vi "Teleop.vi"(10 "Match Info":T1={"Autonomous Elapsed Seconds"=0.0, "TeleOp Elapsed Seconds"=0.0, "Disabled Elapsed Seconds"=0.0, "Visited Autonomous"=FALSE, "Visited TeleOp"=FALSE, "Visited Disabled"=FALSE, "Autonomous Settings"={"Autonomous Style"=enum."Independent", "VI Refnum"=refnum}}, 11 "Call Context":T2) -> ()   [LabVIEW 2013]
doc: "This VI is called for each TeleOp packet received from the DS where the robot is not disabled. It is often used to read from the joysticks and update I/O or to update setpoints for timed control loops. It should complete and return within 20 milliseconds or it may miss DS packets."
uses:
  <vilib>/Rock Robotics/WPI/DriverStation/WPI_DriverStationDerivedRobotMode.ctl
  <vilib>/Rock Robotics/WPI/DriverStation/WPI_DriverStationMatch Info.ctl
  Robot Global Data.vi
  <vilib>/Rock Robotics/WPI/Solenoid/Deprecated/WPI_SolenoidSetBool.vi
  <vilib>/Rock Robotics/WPI/Joystick/WPI_JoystickGetSetRefNum.vi
  <vilib>/Rock Robotics/WPI/Solenoid/Deprecated/WPI_SolenoidGetBool.vi
  <vilib>/Rock Robotics/WPI/RobotDrive/WPI_RobotDriveGetSetRefNum.vi
panel:
  in  "Shoulder Limit":dbl=5.0
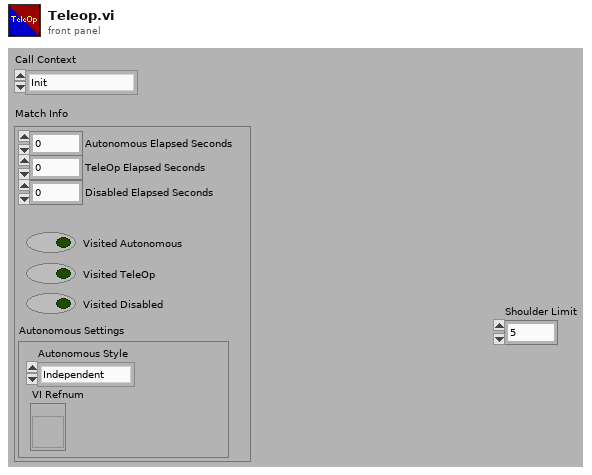
[diagram p1: front panel]
types:
  T1 = typedef "WPI_DriverStationMatch Info.ctl" = cluster{"Autonomous Elapsed Seconds":dbl, "TeleOp Elapsed Seconds":dbl, "Disabled Elapsed Seconds":dbl, "Visited Autonomous":bool, "Visited TeleOp":bool, "Visited Disabled":bool, "Autonomous Settings":cluster{"Autonomous Style":enum16{"Iterative", "Independent"}, "VI Refnum":refnum<vi>}}
  T2 = typedef "WPI_DriverStationDerivedRobotMode.ctl" = enum16{"Init", "Execute", "Stop"}
  T3 = typedef "WPI_JoystickDevRef.ctl" = cluster{"Device":T4}
  T4 = typedef "WPI_JoystickDeviceEnum.ctl" = enum16{"USB 1", "USB 2", "USB 3", "USB 4", "Kinect 1", "Kinect 2"}
  T5 = typedef "WPI_RobotDriveDevRef.ctl" = cluster{"DevStatus":errorcluster, "Motors[]":T6[], "Square Inputs":bool, "Max Output":dbl, "Isochronous":bool}
  T6 = typedef "WPI_MotorControlDeviceRef.ctl" = cluster{"DeviceStatus":errorcluster, "Type":enum16{"PWM", "CAN"}, "PWM":cluster{"Digital Module":T7, "PWM Channel":T8, "DeadBand":T9}, "CAN":cluster{"Device Number":u8, "Control Mode":T10, "Semaphore":T11, "Max Vout":dbl}, "Invert":bool, "TransformRef":T12, "InvTransformRef":T12}
  T7 = typedef "FPGA_TypedefDigitalModule.ctl" = enum16{"Digital Module 1", "Digital Module 2"}
  T8 = typedef "FPGA_DIOPWMChannel.ctl" = enum8{"PWM 1", "PWM 2", "PWM 3", "PWM 4", "PWM 5", "PWM 6", "PWM 7", "PWM 8", "PWM 9", "PWM 10", "Invalid"}
  T9 = typedef "WPI_PWMDeadband.ctl" = cluster{"Name":string, "maxPositivePwm":i32, "minPositivePwm":i32, "centerPwm":i32, "maxNegativePwm":i32, "minNegativePwm":i32, "angularRange":u16}
  T10 = typedef "WPI_CANJaguar_ControlMode.ctl" = enum8{"Percent VBus", "Current", "Speed", "Position", "Voltage"}
  T11 = typedef "Semaphore RefNum" = refnum<k1>
  T12 = typedef "WPI_PWMTransform_ConPane.ctl" = refnum<vi>
  T13 = typedef "WPI_JoystickButtonState.ctl" = cluster{"Button 1":bool, "Button 2":bool, "Button 3":bool, "Button 4":bool, "Button 5":bool, "Button 6":bool, "Button 7":bool, "Button 8":bool, "Button 9":bool, "Button 10":bool, "Button 11":bool, "Button 12":bool}
  T14 = cluster{"axis 1 (x)":dbl, "axis 2 (y)":dbl, "axis 3 (throttle)":dbl, "axis 4":dbl, "axis 5":dbl, "axis 6":dbl}
  T15 = typedef "WPI_SolenoidDevRef.ctl" = cluster{"DevStatus":errorcluster, "Solenoid Module":T16, "Forward Solenoid Channel":T17, "Reverse Solenoid Channel":T17}
  T16 = typedef "FPGA_TypedefSolenoidModule.ctl" = enum16{"Solenoid Module 1", "Solenoid Module 2"}
  T17 = typedef "WPI_SolenoidChannel.ctl" = enum8{"Solenoid 1", "Solenoid 2", "Solenoid 3", "Solenoid 4", "Solenoid 5", "Solenoid 6", "Solenoid 7", "Solenoid 8", "Invalid"}
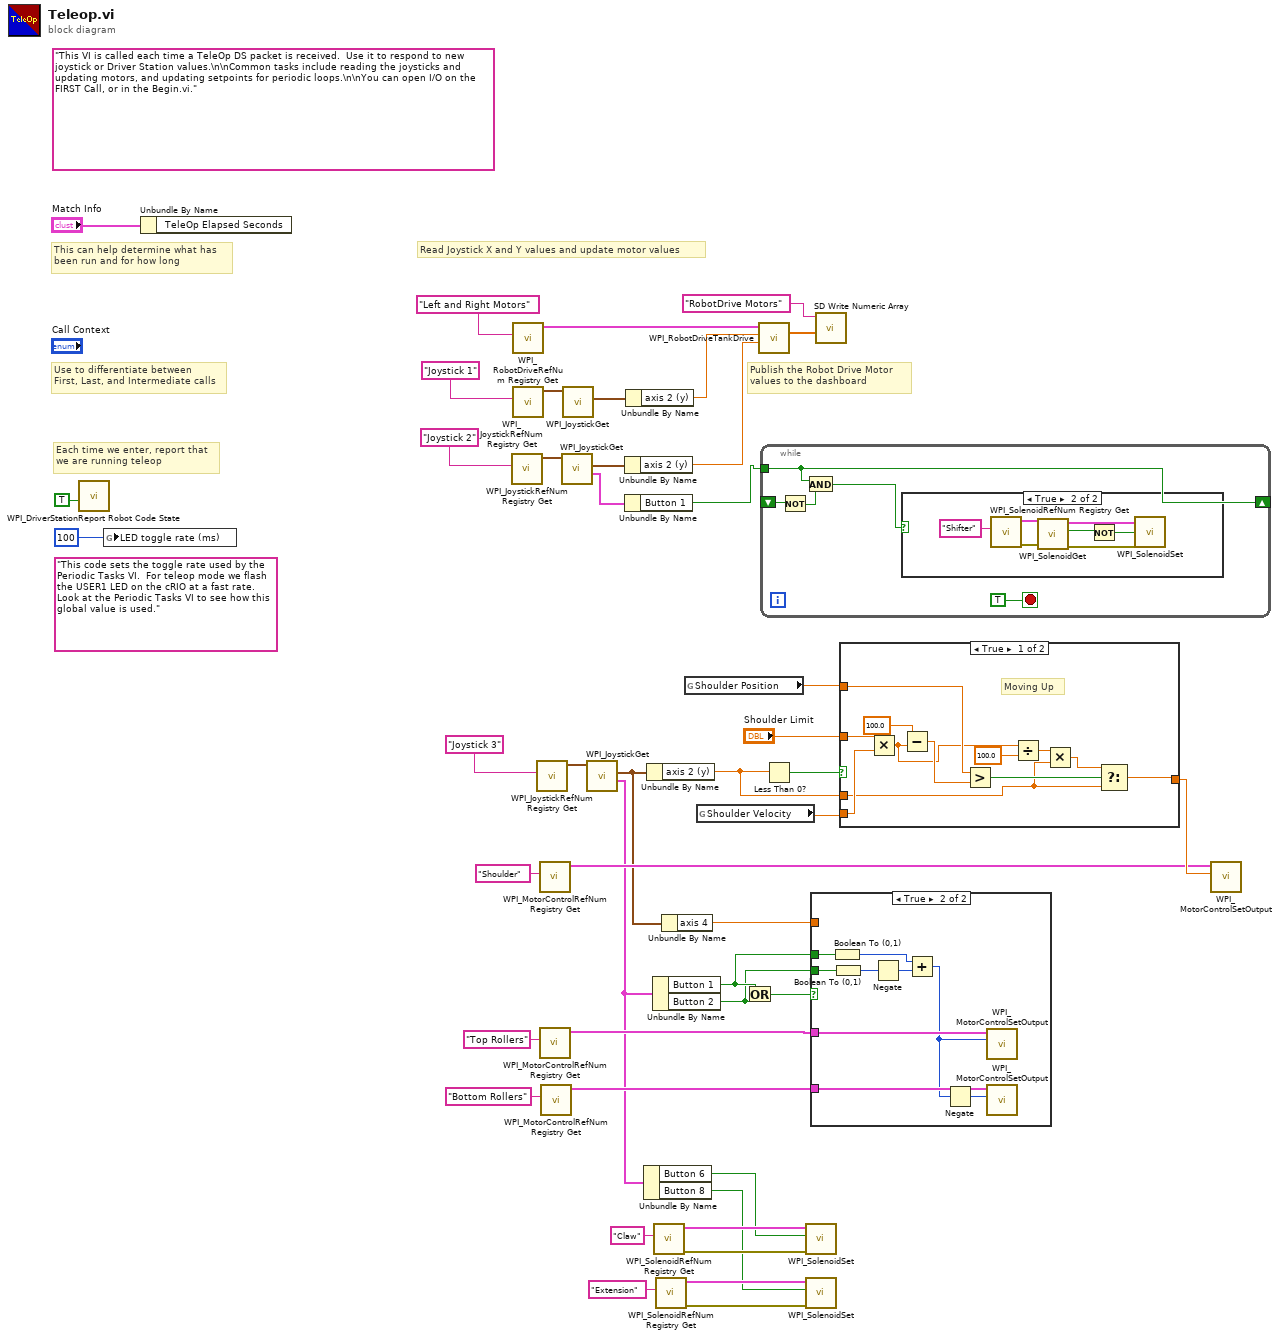
[diagram p0: block diagram]
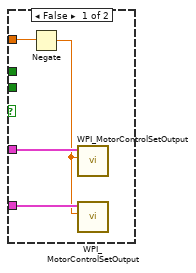
[diagram p3: hidden frame]
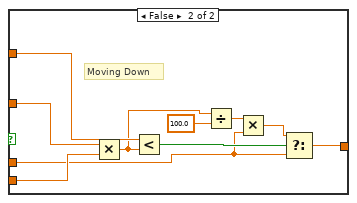
[diagram p4: hidden frame]
diagram:
  (unwired) "This code sets the toggle rate used by the Periodic Tasks VI.  For teleop mode we flash the USER1 LED on the cRIO at a fast rate.  Look at the Periodic Tasks VI to see how this global value is used."
  (unwired) "This VI is called each time a TeleOp DS packet is received.  Use it to respond to new joystick or Driver Station values.\n\nCommon tasks include reading the joysticks and updating motors, and updating setpoints for periodic loops.\n\nYou can open I/O on the FIRST Call, or in the Begin.vi."
  # "Publish the Robot Drive Motor\nvalues to the dashboard"
  # "Each time we enter, report that\nwe are running teleop"
  # "Use to differentiate between\nFirst, Last, and Intermediate calls"
  # "This can help determine what has\nbeen run and for how long"
  # "Read Joystick X and Y values and update motor values"
  n1 = call <vilib>:"WPI_DriverStationReport Robot Code State.vi"("TeleOp"=TRUE ("Autonomous")) -> ()  [unwired: 10 in, 1 out]
  n2 = global write "Robot Global Data.vi" "LED toggle rate (ms)"(u32 100 ("LED ms toggle rate")) -> ()
  n3 = Unbundle By Name("Match Info") -> ()  [unwired: 1 out]
  n4 = call <vilib>:"WPI_JoystickRefNum Registry Get.vi"("refnum name"="Joystick 2") -> ("JoystickDevRef"=w33:T3)  [unwired: 1 in, 9 out]
  n5 = call <vilib>:"WPI_RobotDriveRefNum Registry Get.vi"("refnum name"="Left and Right Motors") -> ("RobotDriveDevRef"=w43:T5)  [unwired: 1 in, 9 out]
  n6 = call <vilib>:"WPI_JoystickRefNum Registry Get.vi"("refnum name"="Joystick 1") -> ("JoystickDevRef"=w40:T3)  [unwired: 1 in, 9 out]
  n7 = call <vilib>:"WPI_JoystickRefNum Registry Get.vi"("refnum name"="Joystick 3") -> ("JoystickDevRef"=w28:T3)  [unwired: 1 in, 9 out]
  n8 = call <vilib>:"WPI_MotorControlRefNum Registry Get.vi"("refnum name"="Shoulder") -> ("MotorControlDevRef"=w20:T6)  [unwired: 9 in, 1 out]
  n9 = call <vilib>:"WPI_MotorControlRefNum Registry Get.vi"("refnum name"="Top Rollers") -> ("MotorControlDevRef"=w14:T6)  [unwired: 9 in, 1 out]
  n10 = call <vilib>:"WPI_MotorControlRefNum Registry Get.vi"("refnum name"="Bottom Rollers") -> ("MotorControlDevRef"=w13:T6)  [unwired: 9 in, 1 out]
  n11 = call <vilib>:"WPI_JoystickGet.vi"("JoystickDevRef"=w33) -> ("Buttons"=w30:T13, "Axes"=w32:T14)  [unwired: 1 in, 4 out]
  n12 = call <vilib>:"WPI_JoystickGet.vi"("JoystickDevRef"=w40) -> ("Axes"=w37:T14)  [unwired: 1 in, 5 out]
  n13 = call <vilib>:"WPI_JoystickGet.vi"("JoystickDevRef"=w28) -> ("Buttons"=w4:T13, "Axes"=w19:T14)  [unwired: 1 in, 4 out]
  n14 = Unbundle By Name(w32) -> ("axis 2 (y)"=w31:dbl)
  n15 = Unbundle By Name(w30) -> ("Button 1"=w1:bool)
  n16 = Unbundle By Name(w37) -> ("axis 2 (y)"=w42:dbl)
  n17 = Unbundle By Name(w4) -> ("Button 6"=w3:bool, "Button 8"=w2:bool)
  n18 = Unbundle By Name(w19) -> ("axis 2 (y)"=w25:dbl)
  n19 = Unbundle By Name(w4) -> ("Button 1"=w12:bool, "Button 2"=w11:bool)
  n20 = call <vilib>:"WPI_SolenoidRefNum Registry Get.vi"("refnum name"="Claw") -> ("error out"=w10:errorcluster, "SolenoidDevRef"=w9:T15)  [unwired: 9 in]
  n21 = call <vilib>:"WPI_SolenoidRefNum Registry Get.vi"("refnum name"="Extension") -> ("error out"=w7:errorcluster, "SolenoidDevRef"=w6:T15)  [unwired: 9 in]
  n22 = Unbundle By Name(w19) -> ("axis 4"=w15:dbl)
  n23 = global read "Robot Global Data.vi" "Shoulder Position"() -> (w24:dbl)
  n24 = global read "Robot Global Data.vi" "Shoulder Velocity"() -> (w23:dbl)
  n25 = Or(x=w12, y=w11) -> (x .or. y?=w18:bool)
  n26 = call <vilib>:"WPI_RobotDriveTankDrive.vi"("Right axis value"=w31, "Left axis value"=w42, "RobotDriveDevRef"=w43) -> ("Motor Values"=w35:dbl[])  [unwired: 6 in, 2 out]
  n27 = while {
    shift-right: [w49] -> _
    shift-left: _ -> [w50]
    tunnel: w1 -> [w49]
    stop <- TRUE stop-if-true
    n28 = Not(x=w50) -> (.not. x?=w48:bool)
    n29 = And(x=w49, y=w48) -> (x .and. y?=w46:bool)
    n30 = case shown="True" w46 {
      frame False {
      }
      frame True {
        n31 = call <vilib>:"WPI_SolenoidRefNum Registry Get.vi"("refnum name"="Shifter") -> ("error out"=w56:errorcluster, "SolenoidDevRef"=w55:T15)  [unwired: 9 in]
        n32 = call-poly <vilib>:"WPI_SolenoidGet.vi"("error in (no error)"=w56, "SolenoidDevRef"=w55) -> ("error out"=w51:errorcluster, "Value"=w54:bool, "SolenoidDevRef"=w52:T15)  [unwired: 7 in]
        n33 = Not(x=w54) -> (.not. x?=w53:bool)
        n34 = call-poly <vilib>:"WPI_SolenoidSet.vi"("error in (no error)"=w51, "Value"=w53, "SolenoidDevRef"=w52) -> ()  [unwired: 7 in, 2 out]
      }
    }
  }
  n35 = Less Than 0?(x=w25) -> (x < 0?=w27:bool)
  n36 = call-poly <vilib>:"WPI_SolenoidSet.vi"("error in (no error)"=w10, "Value"=w3, "SolenoidDevRef"=w9) -> ()  [unwired: 7 in, 2 out]
  n37 = call-poly <vilib>:"WPI_SolenoidSet.vi"("error in (no error)"=w7, "Value"=w2, "SolenoidDevRef"=w6) -> ()  [unwired: 7 in, 2 out]
  n38 = case shown="True" w18 {
    tunnel: w15 -> [w61 _]
    tunnel: w14 -> [w60 w65]
    tunnel: w13 -> [w59 w64]
    tunnel: w12 -> [_ w67]
    tunnel: w11 -> [_ w66]
    frame False {
      n39 = Negate(x=w61) -> (-x=w58:dbl)
      n40 = call <vilib>:"WPI_MotorControlSetOutput.vi"("Output"=w58, "MotorControlDevRef"=w60) -> ()  [unwired: 7 in, 3 out]
      n41 = call <vilib>:"WPI_MotorControlSetOutput.vi"("Output"=w58, "MotorControlDevRef"=w59) -> ()  [unwired: 7 in, 3 out]
    }
    frame True {
      n42 = Boolean To (0,1)(Boolean=w67) -> (0, 1=w68:i16)
      n43 = Boolean To (0,1)(Boolean=w66) -> (0, 1=w70:i16)
      n44 = Negate(x=w70) -> (-x=w69:i16)
      n45 = Add(x=w68, y=w69) -> (x+y=w63:i16)
      n46 = Negate(x=w63) -> (-x=w62:i16)
      n47 = call <vilib>:"WPI_MotorControlSetOutput.vi"("Output"=w63, "MotorControlDevRef"=w65) -> ()  [unwired: 7 in, 3 out]
      n48 = call <vilib>:"WPI_MotorControlSetOutput.vi"("Output"=w62, "MotorControlDevRef"=w64) -> ()  [unwired: 7 in, 3 out]
    }
  }
  n49 = call <vilib>:"SD Write Numeric Array.vi"("Numeric Array"=w35, "Name"="RobotDrive Motors") -> ()  [unwired: 8 in, 2 out]
  n50 = case shown="True" w27 {
    tunnel: w24 -> [w81 w91]
    tunnel: w25 -> [w74 w85]
    tunnel: [w80 w90] -> w21
    tunnel: w23 -> [w78 w89]
    tunnel: "Shoulder Limit" -> [w79 w88]
    frame True {
      # "Moving Up"
      n51 = Multiply(x=w79, y=w78) -> (x*y=w72:dbl)
      n52 = Subtract(x=100.0, y=w72) -> (x-y=w76:dbl)
      n53 = Greater?(x=w81, y=w76) -> (0:w82:bool)
      n54 = Divide(x=w72, y=100.0) -> (x/y=w73:dbl)
      n55 = Multiply(x=w73, y=w74) -> (x*y=w75:dbl)
      n56 = Select(t=w75, s=w82, f=w74) -> (s? t:f=w80:dbl)
    }
    frame False {
      # "Moving Down"
      n57 = Multiply(x=w88, y=w89) -> (x*y=w83:dbl)
      n58 = Less?(x=w91, y=w83) -> (x < y?=w92:bool)
      n59 = Divide(x=w83, y=100.0) -> (x/y=w86:dbl)
      n60 = Multiply(x=w86, y=w85) -> (x*y=w84:dbl)
      n61 = Select(t=w84, s=w92, f=w85) -> (s? t:f=w90:dbl)
    }
  }
  n62 = call <vilib>:"WPI_MotorControlSetOutput.vi"("Output"=w21, "MotorControlDevRef"=w20) -> ()  [unwired: 7 in, 3 out]
